vi "Get Diverter Port.vi"(8 "error in (no error)":errorcluster, 11 "VISA resource name":refnum<visa-resource-name>) -> (0 "error out":errorcluster, 2 "Diverter Port":T1, 3 "VISA resource name out":refnum<visa-resource-name>, 4 "read buffer":string)   [LabVIEW 2019, in "SpectraPro.lvlib"]
uses:
  SpectraPro.lvlib
  Types/Diverter Port.ctl
panel:
  out "output 2":string
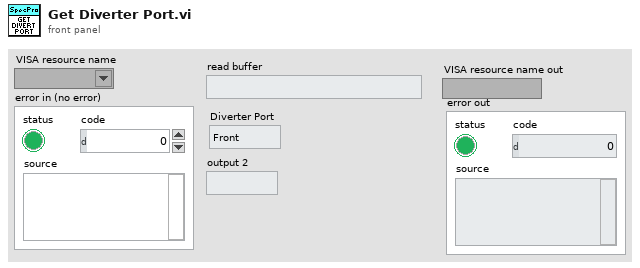
[diagram p1: front panel]
types:
  T1 = typedef "SpectraPro.lvlib/Diverter Port.ctl" = enum16{"Front", "Side"}
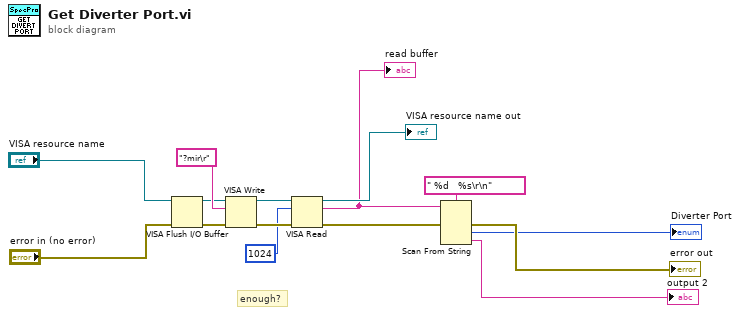
[diagram p0: block diagram]
diagram:
  # "enough?"
  n1 = VISA Flush I/O Buffer(VISA resource name="VISA resource name", error in (no error)="error in (no error)") -> (VISA resource name out=w3:refnum<visa-resource-name>, error out=w5:errorcluster)  [unwired: 1 in]
  n2 = VISA Write(VISA resource name=w3, write buffer="?mir\r", error in (no error)=w5) -> (VISA resource name out=w13:refnum<visa-resource-name>, error out=w14:errorcluster)  [unwired: 1 out]
  n3 = VISA Read(VISA resource name=w13, byte count=u32 1024, error in (no error)=w14) -> (VISA resource name out=→"VISA resource name out":refnum<visa-resource-name>, read buffer=w6:string, error out=w7:errorcluster)  [unwired: 1 out]
  "read buffer" <- w6
  n4 = Scan From String(format string=" %d   %s\r\n", input string=w6, error in=w7) -> (error out=→"error out":errorcluster, output 1=→"Diverter Port":T1, output 2=→"output 2":string)  [unwired: 3 in, 2 out]
